vi "Receive.vi"(8 "error in (no error)":errorcluster, 10 "Transfer Group in":refnum<class "Transfer Group.lvclass">, 11 "UDP Transceiver in":refnum<class "UDP Transceiver.lvclass">) -> (0 "error out":errorcluster, 2 "Transfer Group out":refnum<class "Transfer Group.lvclass">, 3 "UDP Transceiver out":refnum<class "UDP Transceiver.lvclass">)   [LabVIEW 2017, in "UDP.lvlib" / "UDP Transceiver.lvclass"]
uses:
  UDP Transceiver.lvclass
  Builds/Data Sharing Framework/Current/Data Sharing Framework Core/DSF Core.lvlibp/Engine/Classes/Transfer Group/Transfer Group.lvclass
  UDP Transceiver.lvclass/UDP Transceiver.ctl
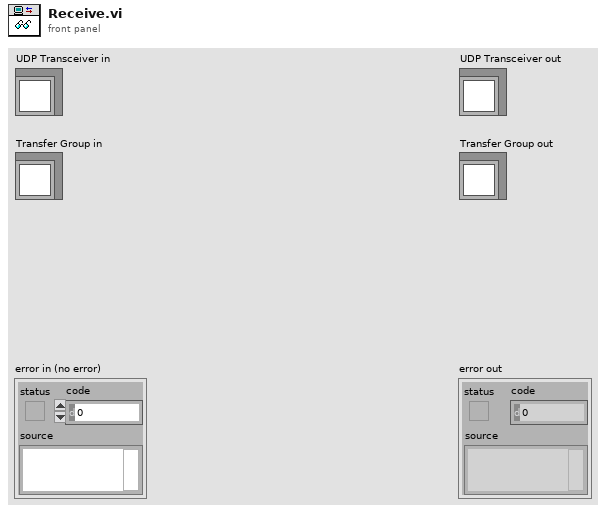
[diagram p1: front panel]
types:
  T1 = typedef "UDP.lvlib/UDP Transceiver.lvclass/Transfer Group Parameters.ctl" = cluster{"Rx":T2, "Tx":T4}
  T2 = typedef "UDP.lvlib/UDP Transceiver.lvclass/Transfer Group Rx Parameters.ctl" = cluster{"Transfers Rx":T3[], "max size":i32}
  T3 = typedef "UDP.lvlib/UDP Transceiver.lvclass/Transfer Rx Parameters.ctl" = cluster{"timeout":i32, "source address":u32, "source port":u16}
  T4 = typedef "UDP.lvlib/UDP Transceiver.lvclass/Transfer Group Tx Parameters.ctl" = cluster{"Transfers Tx":T5[]}
  T5 = typedef "UDP.lvlib/UDP Transceiver.lvclass/Transfer Tx Parameters.ctl" = cluster{"destination port":u16, "destination address":u32}
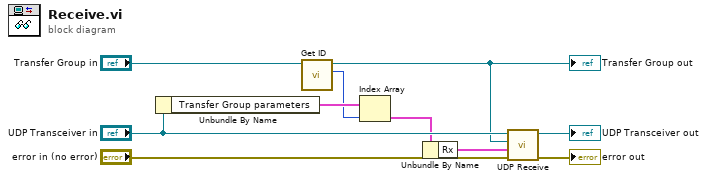
[diagram p0: block diagram]
diagram:
  n1 = Unbundle By Name("UDP Transceiver in") -> ("Transfer Group parameters"=w9:T1[])
  n2 = call "Get ID.vi"("Transfer Group in"="Transfer Group in") -> ("id"=w1:i32, "Transfer Group out"=w2:refnum<class "Transfer Group.lvclass">)  [unwired: 9 in]
  "Transfer Group out" <- w2
  n3 = Index Array(array=w9, index=w1) -> (element=w4:T1)
  n4 = Unbundle By Name(w4) -> ("Rx"=w10:T2)
  n5 = call "UDP Receive.vi"("error in (no error)"="error in (no error)", "Transfer Group Rx parameters"=w10, "Transfer Group"=w2, "UDP Transceiver in"="UDP Transceiver in") -> ("error out"=→"error out":errorcluster, "UDP Transceiver out"=→"UDP Transceiver out":refnum<class "UDP Transceiver.lvclass">)  [unwired: 6 in]
